vi "Air Blast Control.vi"(8 "error in (no error)":errorcluster, 9 "Enable Heater (F)":bool, 10 "Enable Air Flow (F)":bool) -> (0 "error out":errorcluster)   [LabVIEW 2010]
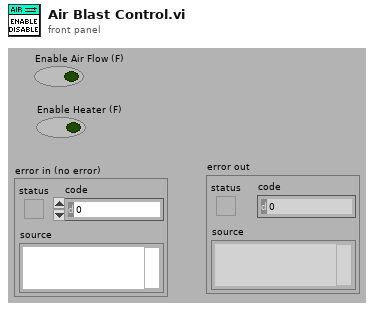
[diagram p1: front panel]
types:
  T1 = enum16{"--Disconnect All--", "Connect PulseGen to CH1", "Connect PulseGen to CH2", "Connect PulseGen to CH3", "Connect PulseGen to CH4", "Connect PulseGen to CH5", "Connect PulseGen to CH6", "Connect PulseGen to CH7", "Connect PulseGen to CH8", "Connect PulseGen to CH9", "Connect PulseGen to CH10", "Connect PulseGen to CH11", "Connect PulseGen to CH12", "Connect PulseGen to CH13", "Connect PulseGen to CH14", "Connect PulseGen to CH15", "Connect PulseGen to CH16", "Connect PulseGen to CH17", "Connect PulseGen to CH18", "Connect PulseGen to CH19", "Connect PulseGen to CH20", "Connect PulseGen to CH21", "Connect PulseGen to CH22", "Connect PulseGen to CH23", "Connect PulseGen to CH24", "Connect PulseGen to CH25", "Set MAG_SW", "Set Dynamic Load", "Set Expansion Trigger", "Trigger Positive Pulse", "Trigger Negative Pulse", "Set MSP Magic Pin", "Set BAT_EN", "Connect MSP_ACLK to CTR", "Connect MSP_MCLK to CTR", "Connect MSP_DIG_TST_OUT to CTR", "Connect STIM_SCK to CTR", "Connect STIM_CLK to CTR", "Connect SMU2 to Magnet", "Magnet Enable", "Cap Short", "Connect Positive Pulse to Pulse Bus", "Connect Negative Pulse to Pulse Bus", "Connect JTAG", "Connect JTAG DVDD Power", "RF Attach", "Connect SMU3 to VBAT", "Connect SMU3 Soft Start", "Connect ARB to Charge Coil", "Connect ARB to Matrix", "Connect CTR to Matrix", "DMM_I Short", "DMM_I 1000 Ohm", "DMM_I 100 Ohm", "DMM_I 10 Ohm", "Connect CH25 to DUT GND", "Enclosure Lights", "Heat Fan Zone 1", "Heat Fan Zone 2", "Temp Zone 1", "Temp Zone 2", "Temp Zone 3", "Guard Door Locks", "Air Heat Zone 3", "Zone 3 Vent", "Zone 3 Loader", "Zone 3 Upper Bed", "Zone 3 Lower Bed", "Zone 3 Standby Temp", "Yellow Light", "Red Light", "Green Light", "Reset Common Test Lines"}
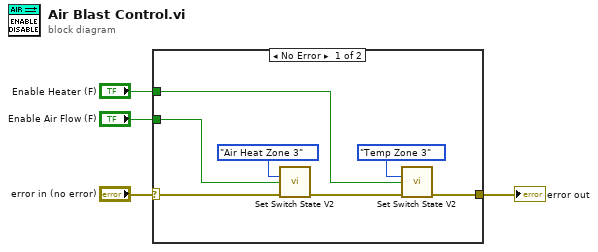
[diagram p0: block diagram]
diagram:
  n1 = case shown="No Error" "error in (no error)" {
    selector: "error in (no error)" -> [w11 w12]
    tunnel: [w5 w12] -> w1
    tunnel: "Enable Air Flow (F)" -> [w9 _]
    tunnel: "Enable Heater (F)" -> [w6 _]
    frame No Error {
      n2 = call "Set Switch State V2.vi"("Action"=T1."Air Heat Zone 3", "State"=w9, "error in (no error)"=w11) -> ("error out"=w8:errorcluster)  [unwired: 12 in]
      n3 = call "Set Switch State V2.vi"("Action"=T1."Temp Zone 3", "State"=w6, "error in (no error)"=w8) -> ("error out"=w5:errorcluster)  [unwired: 12 in]
    }
    frame Error {
    }
  }
  "error out" <- w1
